vi "Demo_2.vi"() -> ()   [LabVIEW 2017]
uses:
  Components/MES_Base.lvlibp/Controls/Test.ctl
  Components/TestView_Base.lvlibp/ViewStatus.ctl
  Components/TestView_Base.lvlibp/TestView_Base.lvclass
  C:/Projects/Client-Audinate/Src/Components/ViPER.lvlibp/ViPER.lvclass
  Components/ViPER.lvlibp/ViPER.lvclass
  Components/MES_Base.lvlibp/MES_Base.lvclass
panel:
  in  "Clear":bool
  in  "DUT":u32
  in  "User":string
  in  "set User":bool
  in  "Status":T1
  in  "set status":bool
  in  "Test":T2={"Code"="", "Name"="", "Description"="", "Group"="", "IsGroup"=FALSE, "Tag"="", "Method"="", "Parrameter"="", "DataType"=enum."String", "Value"=variant, "Status"=enum."Pass", "LimitLo"=variant, "LimitHi"=variant, "StringMatch"="", "BooleanMatch"=FALSE, "DisplayFormat"="", "Units"="", "TestTime"=0.0}
  in  "Set test":bool
  in  "Tests":T2[](array[typedef])
  in  "Set tests":bool
  in  "Title":string
  in  "set title":bool
  in  "SN":string
  in  "set SN":bool
  in  "stop":bool
  in  "Config XML":string="<?xml version=\"1.0\" encoding=\"UTF-8\" standalone=\"no\" ?>\n<Object>\n\n  <Name>TestView</Name>\n\n  <Class>TestView_Tree_Single</Class>\n\n</Object>\n"
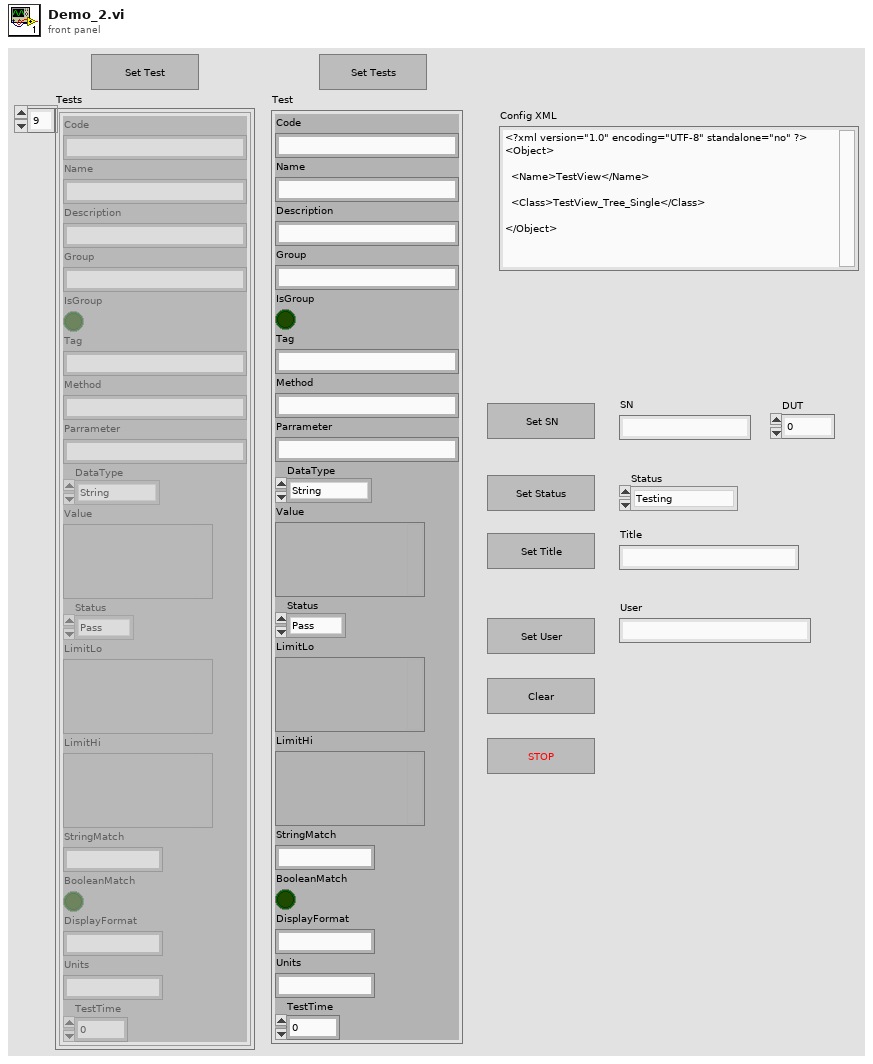
[diagram p1: front panel]
types:
  T1 = typedef "TestView_Base.lvlibp/TestView_Base.lvclass/ViewStatus.ctl" = enum16{"Testing", "Ready", "Logout", "Login", "PASS", "FAIL", "FAULT", "ABORTED"}
  T2 = typedef "MES_Base.lvlibp/MES_Base.lvclass/Test.ctl" = cluster{"Code":string, "Name":string, "Description":string, "Group":string, "IsGroup":bool, "Tag":string, "Method":string, "Parrameter":string, "DataType":enum16{"NA", "String", "Boolean", "Int", "Dbl"}, "Value":variant, "Status":enum16{"Pending", "Pass", "Fail"}, "LimitLo":variant, "LimitHi":variant, "StringMatch":string, "BooleanMatch":bool, "DisplayFormat":string, "Units":string, "TestTime":dbl}
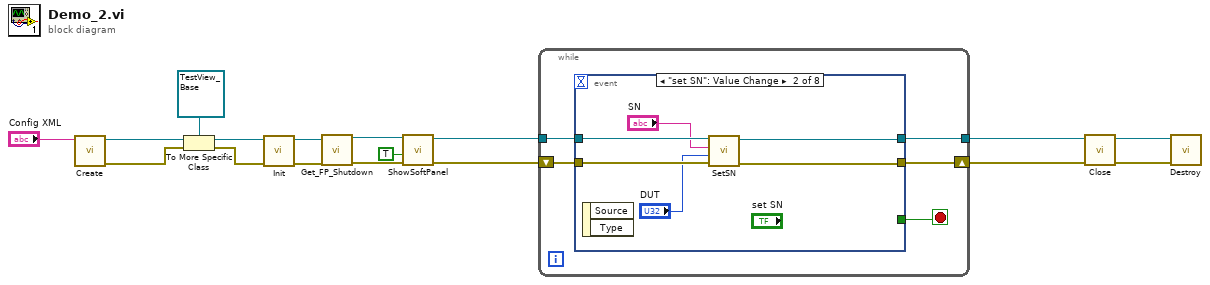
[diagram p0: block diagram]
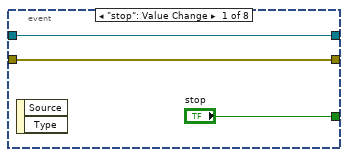
[diagram p2: hidden frame]
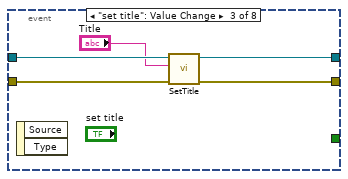
[diagram p3: hidden frame]
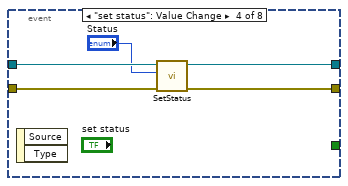
[diagram p4: hidden frame]
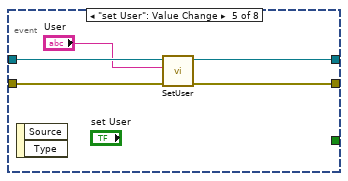
[diagram p5: hidden frame]
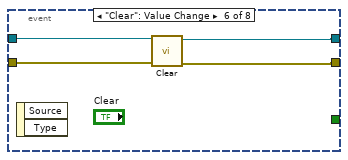
[diagram p6: hidden frame]
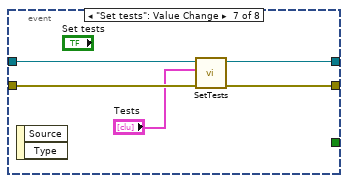
[diagram p7: hidden frame]
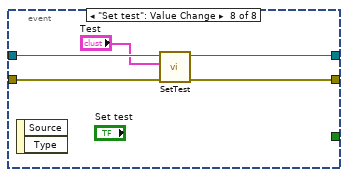
[diagram p8: hidden frame]
diagram:
  n1 = call "Create.vi"("Config XML"="Config XML") -> ("error out"=w6:errorcluster, "reference out"=w4:refnum<class "ViPER.lvclass">)  [unwired: 9 in]
  n2 = To More Specific Class(target class=refnum<class "TestView_Base.lvclass"> refnum ("TestView_Base.lvlibp:TestView_Tree"), reference=w4, error in=w6) -> (specific class reference=w3:refnum<class "TestView_Base.lvclass">, error out=w5:errorcluster)
  n3 = call-dynamic "Init.vi"("error in (no error)"=w5, "reference in"=w3) -> ("error out"=w16:errorcluster, "reference in"=w15:refnum<class "TestView_Base.lvclass">)  [unwired: 8 in]
  n4 = call "Get_FP_Shutdown.vi"("ViKing_Base in"=w15, "error in (no error)"=w16) -> ("ViKing_Base out"=w13:refnum<class "TestView_Base.lvclass">, "error out"=w14:errorcluster)  [unwired: 9 in, 3 out]
  n5 = call-dynamic "ShowSoftPanel.vi"("error in (no error)"=w14, "Floating"=TRUE, "Driver in"=w13) -> ("error out"=w1:errorcluster, "Driver out"=w2:refnum<class "TestView_Base.lvclass">)  [unwired: 6 in, 1 out]
  n6 = while {
    tunnel: w2 -> [w21]
    shift-right: [w19] -> w9
    shift-left: w1 -> [w22]
    tunnel: [w18] -> w10
    stop <- w20 stop-if-true
    n7 = event shown="[1] \"set SN\": Value Change" {
      selector: _ -> [_ _ _ _ _ _ _ _]
      dyn-events: _ -> [_ _ _ _ _ _ _ _]
      timeout: _ -> [_ _ _ _ _ _ _ _]
      tunnel: w22 -> [w24 w31 w36 w41 w46 w50 w55 w60]
      tunnel: w21 -> [w23 w30 w35 w40 w45 w49 w53 w59]
      tunnel: ["stop" _ _ _ _ _ _ _] -> w20
      tunnel: [w24 w29 w34 w39 w44 w48 w54 w58] -> w19
      tunnel: [w23 w28 w33 w38 w43 w47 w52 w57] -> w18
      event "stop": Value Change {
        n8 = event-data() -> ()  [unwired: 1 in, 2 out]
      }
      event "set SN": Value Change {
        n9 = event-data() -> ()  [unwired: 1 in, 2 out]
        n10 = call-dynamic "SetSN.vi"("error in (no error)"=w31, "DUT"="DUT", "SN"="SN", "reference in"=w30) -> ("error out"=w29:errorcluster, "reference in"=w28:refnum<class "TestView_Base.lvclass">)  [unwired: 6 in]
      }
      event "set title": Value Change {
        n11 = event-data() -> ()  [unwired: 1 in, 2 out]
        n12 = call-dynamic "SetTitle.vi"("error in (no error)"=w36, "Title"="Title", "reference in"=w35) -> ("error out"=w34:errorcluster, "reference in"=w33:refnum<class "TestView_Base.lvclass">)  [unwired: 7 in]
      }
      event "set status": Value Change {
        n13 = event-data() -> ()  [unwired: 1 in, 2 out]
        n14 = call-dynamic "SetStatus.vi"("error in (no error)"=w41, "Status"="Status", "reference in"=w40) -> ("error out"=w39:errorcluster, "reference in"=w38:refnum<class "TestView_Base.lvclass">)  [unwired: 7 in]
      }
      event "set User": Value Change {
        n15 = event-data() -> ()  [unwired: 1 in, 2 out]
        n16 = call-dynamic "SetUser.vi"("error in (no error)"=w46, "User"="User", "reference in"=w45) -> ("error out"=w44:errorcluster, "reference in"=w43:refnum<class "TestView_Base.lvclass">)  [unwired: 7 in]
      }
      event "Clear": Value Change {
        n17 = event-data() -> ()  [unwired: 1 in, 2 out]
        n18 = call-dynamic "Clear.vi"("error in (no error)"=w50, "TestView_Tree in"=w49) -> ("error out"=w48:errorcluster, "TestView_Tree out"=w47:refnum<class "TestView_Base.lvclass">)  [unwired: 8 in]
      }
      event "Set tests": Value Change {
        n19 = event-data() -> ()  [unwired: 1 in, 2 out]
        n20 = call-dynamic "SetTests.vi"("error in (no error)"=w55, "Tests"="Tests", "reference in"=w53) -> ("error out"=w54:errorcluster, "reference in"=w52:refnum<class "TestView_Base.lvclass">)  [unwired: 7 in]
      }
      event "Set test": Value Change {
        n21 = event-data() -> ()  [unwired: 1 in, 2 out]
        n22 = call-dynamic "SetTest.vi"("error in (no error)"=w60, "Test"="Test", "reference in"=w59) -> ("error out"=w58:errorcluster, "reference in"=w57:refnum<class "TestView_Base.lvclass">)  [unwired: 7 in]
      }
    }
  }
  n23 = call-dynamic "Close.vi"("error in (no error)"=w9, "reference in"=w10) -> ("error out"=w12:errorcluster, "reference in"=w11:refnum<class "TestView_Base.lvclass">)  [unwired: 8 in]
  n24 = call "Destroy.vi"("error in (no error)"=w12, "reference in"=w11) -> ()  [unwired: 9 in, 1 out]
